vi "segToPoints.vi"(11 "Line Segment":T1) -> (3 "points":cluster{"X":sgl, "Y":sgl}[](array[cluster]))   [LabVIEW 2015]
uses:
  <vilib>/vision/NI_Vision_Development_Module.lvlib
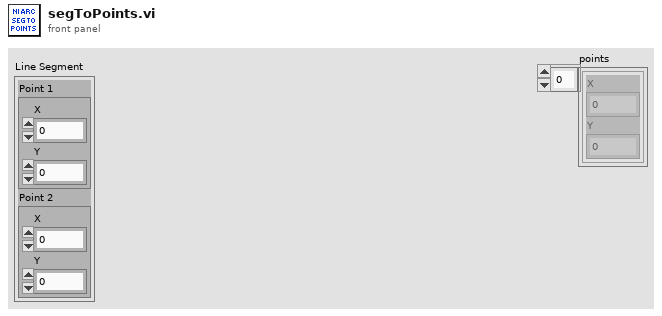
[diagram p1: front panel]
types:
  T1 = cluster{"Point 1":cluster{"X":sgl, "Y":sgl}, "Point 2":cluster{"X":sgl, "Y":sgl}}
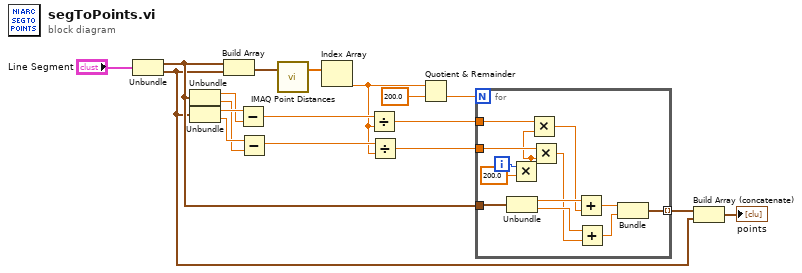
[diagram p0: block diagram]
diagram:
  n1 = Unbundle("Line Segment") -> ("Point 1"=w4:cluster{"X":sgl, "Y":sgl}, "Point 2"=w2:cluster{"X":sgl, "Y":sgl})
  n2 = Unbundle(w4) -> ("X"=w13:sgl, "Y"=w11:sgl)
  n3 = Unbundle(w2) -> ("X"=w14:sgl, "Y"=w12:sgl)
  n4 = Build Array(w4, w2) -> (w18:cluster{"X":sgl, "Y":sgl}[])
  n5 = Subtract(x=w14, y=w13) -> (x-y=w10:sgl)
  n6 = Subtract(x=w12, y=w11) -> (x-y=w9:sgl)
  n7 = call "IMAQ Point Distances"("Points"=w18) -> ("Distances"=w17:sgl[])  [unwired: 4 in, 1 out]
  n8 = Index Array(array=w17) -> (element=w8:sgl)  [unwired: 1 in]
  n9 = Divide(x=w10, y=w8) -> (x/y=w7:sgl)
  n10 = Divide(x=w9, y=w8) -> (x/y=w6:sgl)
  n11 = Quotient & Remainder(x=w8, y=sgl 200.0) -> (floor(x/y)=w5:sgl)  [unwired: 1 out]
  n12 = for {
    N: w5 -> [_]
    tunnel: w7 -> [w31]
    tunnel: w6 -> [w30]
    tunnel: w4 -> [w29]
    tunnel: [w22] -> w3 mode=indexing
    i -> [w21]
    n13 = Unbundle(w29) -> ("X"=w28:sgl, "Y"=w26:sgl)
    n14 = Multiply(x=w21, y=sgl 200.0) -> (x*y=w20:sgl)
    n15 = Multiply(x=w31, y=w20) -> (x*y=w27:sgl)
    n16 = Multiply(x=w30, y=w20) -> (x*y=w25:sgl)
    n17 = Add(x=w28, y=w27) -> (x+y=w24:sgl)
    n18 = Add(x=w26, y=w25) -> (x+y=w23:sgl)
    n19 = Bundle(w24, w23) -> (w22:cluster{sgl, sgl})  [unwired: 1 in]
  }
  n20 = Build Array (concatenate)(w3, w2) -> (→"points":cluster{"X":sgl, "Y":sgl}[])
